vi "fxp.vi"(11 "input":fxp<+/-,64,32>) -> (3 "output":fxp<+/-,64,33>)   [LabVIEW 2020]
panel:
  in  "in2":dbl
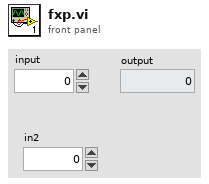
[diagram p1: front panel]
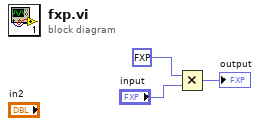
[diagram p0: block diagram]
diagram:
  n1 = Multiply(x=fxp<+,1,2> 2.0, y="input") -> (x*y=→"output":fxp<+/-,64,33>)
